vi "getResults.vi"(8 "error in (no error)":errorcluster, 11 "Instrument.LockinAPI in":refnum<class "Instrument.LockinAPI.lvclass">) -> (0 "error out":errorcluster, 1 "Time Stamp":timestamp, 2 "Results (Dictionary)":cluster{"key":string, "value":dbl}[](array[cluster]), 3 "Instrument.LockinAPI out":refnum<class "Instrument.LockinAPI.lvclass">)   [LabVIEW 2019, in "Instrument.LockinAPI.lvclass"]
doc: "API to get the results of lockin calculation.\n\nIf address=\"\", this API reads from localhost\nIf address is remote lockin, you need to add this computer to allowed whitelist on the lockin computer you are trying to access."
uses:
  Instrument.LockinAPI.lvclass
  C:/Users/patrick/Documents/GitHub/Instrument-Framework/lvsrc/Instrument/Instrument.lvclass
  Typedefs/API/LockinAPI.Commands--Enum.ctl
  491cbe65-b421-4c56-8bbf-cf37146840a5.vi
  491cbe65-b421-4c56-8bbf-cf37146840a5.vi/7e5d1003-cfc7-45d4-8f33-8ca952ae8cb3.vi
  491cbe65-b421-4c56-8bbf-cf37146840a5.vi/7e5d1003-cfc7-45d4-8f33-8ca952ae8cb3.vi/5d0563db-fb84-48de-aef4-1e945f8f3f34.vi
  491cbe65-b421-4c56-8bbf-cf37146840a5.vi/7e5d1003-cfc7-45d4-8f33-8ca952ae8cb3.vi/30f9de05-54d1-4e0b-a86c-310425074b4d.vi
  491cbe65-b421-4c56-8bbf-cf37146840a5.vi/7e5d1003-cfc7-45d4-8f33-8ca952ae8cb3.vi/ca2d8494-89d4-4ca0-b4fc-a44a50ba682b.vi
  <vilib>/JDP Science/JSONtext/Make JSON Array.vi
  491cbe65-b421-4c56-8bbf-cf37146840a5.vi/7e5d1003-cfc7-45d4-8f33-8ca952ae8cb3.vi/30f9de05-54d1-4e0b-a86c-310425074b4d.vi/fdfa160c-9e73-4f92-88ec-c064400c872b.vi
  491cbe65-b421-4c56-8bbf-cf37146840a5.vi/7e5d1003-cfc7-45d4-8f33-8ca952ae8cb3.vi/ca2d8494-89d4-4ca0-b4fc-a44a50ba682b.vi/636c41e2-dda7-456e-9b76-756a1709dba8.vi
  491cbe65-b421-4c56-8bbf-cf37146840a5.vi/7e5d1003-cfc7-45d4-8f33-8ca952ae8cb3.vi/ca2d8494-89d4-4ca0-b4fc-a44a50ba682b.vi/85a596af-4f5c-4423-b741-80276b556a2f.vi
  Instrument/API/Enum to String.vi
  Instrument/Private/Get RC Connection Status.vi
  <vilib>/JDP Science/JSONtext/Variant to JSON Text.vi
  <vilib>/JDP Science/JSONtext/support/Format JSON Array Text.vi
  Instrument/API/Send and Receive.vi
  <vilib>/JDP Science/JSONtext/JSON text to Variant.vi
  <vilib>/Utility/Data Type/Get Type Information.vi
  <vilib>/JDP Science/JSONtext/LVClass Serializer/JSONtext LVClass Serializer.lvclass
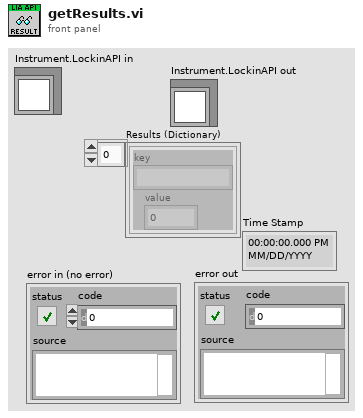
[diagram p1: front panel]
types:
  T1 = cluster{"Time Stamp":timestamp, "Results (Dictionary)":cluster{"key":string, "value":dbl}[]}
  T2 = typedef "Instrument.LockinAPI.lvclass/LockinAPI.Commands--Enum.ctl" = enum16{"setAI", "setAO", "setAO_Amplitude", "setAO_DC", "setAO_Frequency", "setAO_Phase", "setAO_Function", "setAO_I+", "setREF", "setREF_Frequency", "setREF_Phase", "setREF_TC", "setREF_Roll-Off", "setDAQ", "setSampling", "setOffset", "setState", "getState", "getAO", "getAI", "getResults", "getSampling", "getAOconfig", "getREFconfig", "setInputGain", "setOutputGain", "getInputGain", "getOutputGain", "setSamplingMode", "getSamplingMode", "setSweep", "setSweepTime", "setSweepTable", "getStatus", "getSweepResults", "getSweepWaveforms", "startSweep", "stopSweep", "setAUX", "getAUX"}
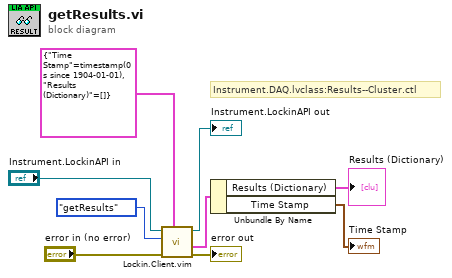
[diagram p0: block diagram]
diagram:
  # "Instrument.DAQ.lvclass:Results--Cluster.ctl"
  n1 = call "Lockin.Client.vim"("Data Out type"=T1 {"Time Stamp"=timestamp(0 s since 1904-01-01), "Results (Dictionary)"=[]} ("input cluster"), "error in (no error)"="error in (no error)", "Command"=LockinAPI.Commands--Enum."getResults", "Instrument.LockinAPI in"="Instrument.LockinAPI in") -> ("error out"=→"error out":errorcluster, "Data out"=w7:T1, "Instrument.LockinAPI out"=→"Instrument.LockinAPI out":refnum<class "Instrument.LockinAPI.lvclass">)  [unwired: 5 in]
  n2 = Unbundle By Name(w7) -> ("Results (Dictionary)"=→"Results (Dictionary)":cluster{"key":string, "value":dbl}[], "Time Stamp"=→"Time Stamp":timestamp)
